vi "test json to variant null.vi"(8 "error in (no error)":errorcluster) -> (0 "error out":errorcluster)   [LabVIEW 2019, in "labview_json_tests.lvlib"]
uses:
  labview_json_tests.lvlib
  lib/labview_json.lvlib
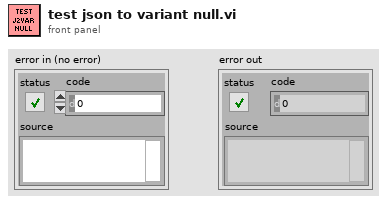
[diagram p1: front panel]
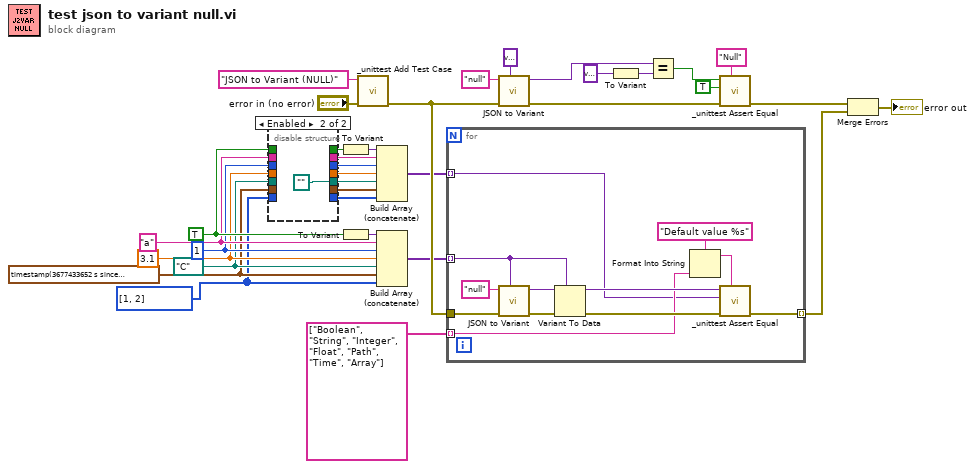
[diagram p0: block diagram]
diagram:
  w9 = i32[] [1, 2]
  w11 = timestamp(3677433652.103939 s since 1904-01-01)
  w13 = path "C:/"
  w15 = 3.1
  w17 = 1
  w19 = "a"
  w21 = TRUE
  n1 = disable-structure shown="Enabled" {
    disable-tunnel: w21 -> [w41 _]
    disable-tunnel: [w41 _] -> w20
    disable-tunnel: w19 -> [w40 _]
    disable-tunnel: [w40 _] -> w18
    disable-tunnel: w17 -> [w39 _]
    disable-tunnel: [w39 _] -> w16
    disable-tunnel: w15 -> [w38 _]
    disable-tunnel: [w38 _] -> w14
    disable-tunnel: w13 -> [w37 _]
    disable-tunnel: [w37 path ""] -> w12
    disable-tunnel: w11 -> [w36 _]
    disable-tunnel: [w36 _] -> w10
    disable-tunnel: w9 -> [w35 _]
    disable-tunnel: [w35 _] -> w8
    frame Disabled {
    }
    frame Enabled {
    }
  }
  n2 = To Variant(anything=w20) -> (Variant=w22:variant)
  n3 = To Variant(anything=w21) -> (Variant=w23:variant)
  n4 = call "_unittest Add Test Case.vi"("error in (no error)"="error in (no error)", "Test Case"="JSON to Variant (NULL)") -> ("error out"=w25:errorcluster)  [unwired: 9 in]
  n5 = Build Array (concatenate)(w22, w18, w16, w14, w12, w10, w8) -> (w6:variant[])
  n6 = Build Array (concatenate)(w23, w19, w17, w15, w13, w11, w9) -> (w7:variant[])
  n7 = for {
    tunnel: w25 -> [w52]
    tunnel: [w51] -> w24 mode=indexing
    tunnel: w7 -> [w48] mode=indexing
    tunnel: w6 -> [w43] mode=indexing
    tunnel: string[] ["Boolean", "String", "Integer", "Float", "Path", "Time", "Array"] -> [w44] mode=indexing
    n8 = call "JSON to Variant.vi"("Variant Type"=w48, "error in (no error)"=w52, "JSON"="null") -> ("error out"=w53:errorcluster, "Variant out"=w49:variant)  [unwired: 7 in]
    n9 = Variant To Data(error in=w53, type=w48, Variant=w49) -> (data=w47:variant, error out=w50:errorcluster)
    n10 = Format Into String(format string="Default value %s" ("Message"), w44) -> (resulting string=w45:string)  [unwired: 2 in, 1 out]
    n11 = call "_unittest Assert Equal.vi"("Message"=w45, "error in (no error)"=w50, "Expected Value"=w43, "Actual Value"=w47) -> ("error out"=w51:errorcluster)  [unwired: 7 in]
  }
  n12 = call "JSON to Variant.vi"("Variant Type"=variant, "error in (no error)"=w25, "JSON"="null") -> ("error out"=w29:errorcluster, "Variant out"=w5:variant)  [unwired: 7 in]
  n13 = To Variant(anything=variant) -> (Variant=w4:variant)
  n14 = Equal?(x=w5, y=w4) -> (x = y?=w3:bool)
  n15 = call "_unittest Assert Equal.vi"("Message"="Null", "error in (no error)"=w29, "Expected Value"=TRUE, "Actual Value"=w3) -> ("error out"=w32:errorcluster)  [unwired: 7 in]
  n16 = Merge Errors(w32, w24) -> (→"error out":errorcluster)
